vi "Untitled-2SubVI (1).vi"(8 "Array in":u16[][](array[numeric]), 9 "Numeric 2":dbl, 10 "Numeric":dbl, 11 "shuffled array":i32[][](array[numeric])) -> (3 "Array out":u16[][](array[numeric]))   [LabVIEW 2020]
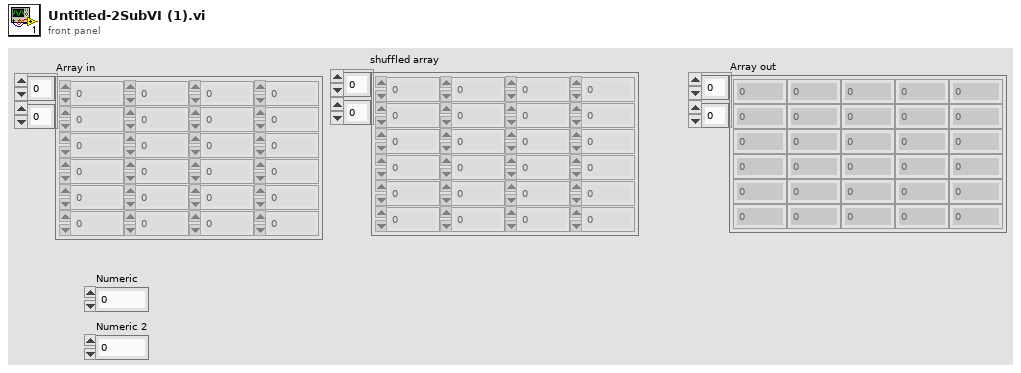
[diagram p1: front panel]
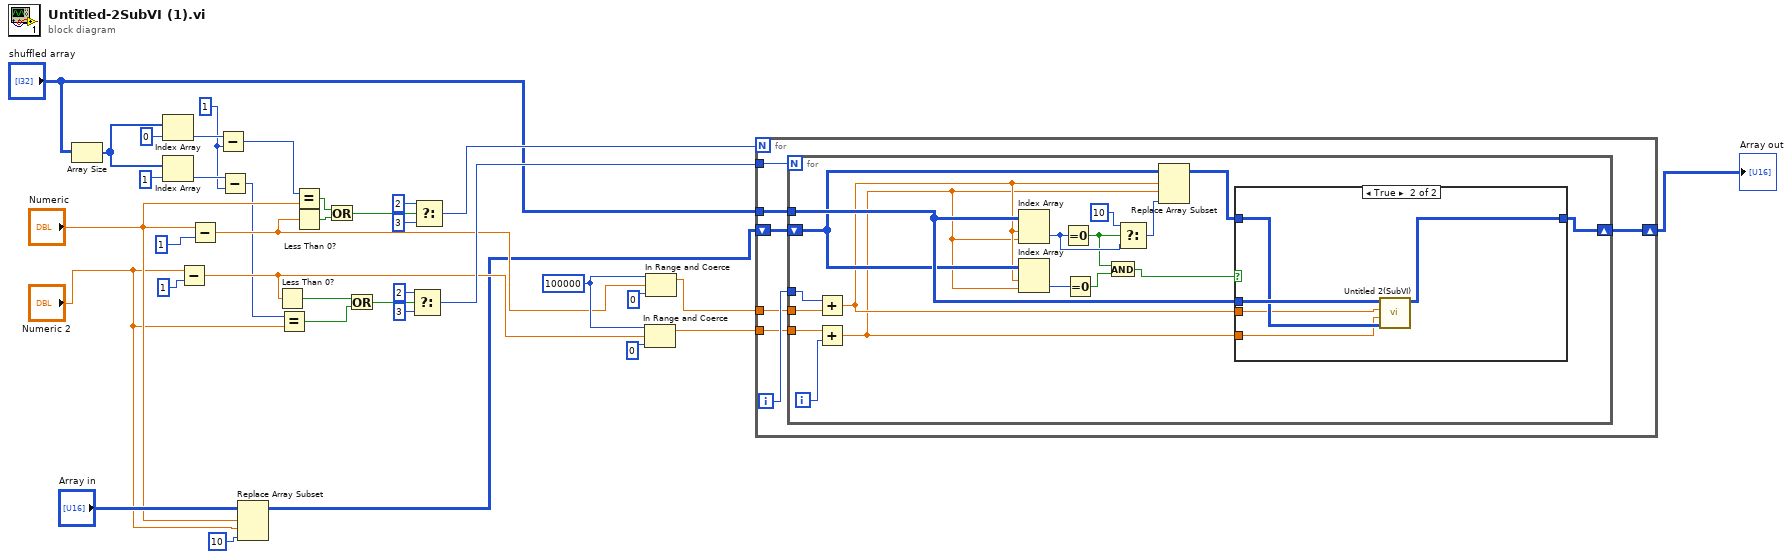
[diagram p0: block diagram]
diagram:
  w3 = 1
  w26 = 100000
  n1 = Array Size(array="shuffled array") -> (size(s)=w16:i32[])
  n2 = Index Array(array=w16, index=0) -> (element=w5:i32)
  n3 = Index Array(array=w16, index=1) -> (element=w4:i32)
  n4 = Subtract(x="Numeric 2", y=1) -> (x-y=w23:dbl)
  n5 = Subtract(x="Numeric", y=1) -> (x-y=w25:dbl)
  n6 = Subtract(x=w5, y=w3) -> (x-y=w2:i32)
  n7 = Subtract(x=w4, y=w3) -> (x-y=w1:i32)
  n8 = Replace Array Subset(array="Array in", new element=10, index (row)="Numeric", index (col)="Numeric 2") -> (w19:u16[][])
  n9 = Less Than 0?(x=w23) -> (x < 0?=w10:bool)
  n10 = Equal?(x=w1, y="Numeric 2") -> (x = y?=w9:bool)
  n11 = Equal?(x=w2, y="Numeric") -> (x = y?=w13:bool)
  n12 = Less Than 0?(x=w25) -> (x < 0?=w14:bool)
  n13 = Or(x=w13, y=w14) -> (x .or. y?=w12:bool)
  n14 = Or(x=w10, y=w9) -> (x .or. y?=w11:bool)
  n15 = Select(t=2, s=w11, f=3) -> (s? t:f=w29:i32)
  n16 = Select(t=2, s=w12, f=3) -> (s? t:f=w30:i32)
  n17 = In Range and Coerce(upper limit=w26, x=w23, lower limit=0) -> (coerced(x)=w21:dbl)  [unwired: 1 out]
  n18 = In Range and Coerce(upper limit=w26, x=w25, lower limit=0) -> (coerced(x)=w22:dbl)  [unwired: 1 out]
  n19 = for {
    N: w30 -> [_]
    tunnel: w29 -> [w42]
    shift-right: [w40] -> w24
    shift-left: w19 -> [w43]
    tunnel: w22 -> [w39]
    tunnel: w21 -> [w38]
    tunnel: "shuffled array" -> [w37]
    i -> [w41]
    n20 = for {
      N: w42 -> [_]
      tunnel: w41 -> [w59]
      shift-right: [w52] -> w40
      shift-left: w43 -> [w50]
      tunnel: w39 -> [w60]
      tunnel: w38 -> [w58]
      tunnel: w37 -> [w51]
      i -> [w57]
      n21 = Add(x=w59, y=w60) -> (x+y=w48:dbl)
      n22 = Add(x=w58, y=w57) -> (x+y=w47:dbl)
      n23 = Index Array(array=w51, index (row)=w48, index (col)=w47) -> (element=w54:i32)
      n24 = Index Array(array=w50, index (row)=w48, index (col)=w47) -> (element=w49:u16)
      n25 = Equal To 0?(x=w54) -> (x = 0?=w45:bool)
      n26 = Equal To 0?(x=w49) -> (x = 0?=w46:bool)
      n27 = And(x=w45, y=w46) -> (x .and. y?=w44:bool)
      n28 = Select(t=10, s=w45, f=w54) -> (s? t:f=w56:i32)
      n29 = Replace Array Subset(array=w50, new element=w56, index (row)=w48, index (col)=w47) -> (w53:u16[][])
      n30 = case shown="True" w44 {
        tunnel: w53 -> [w61 w65]
        tunnel: [w61 w64] -> w52
        tunnel: w51 -> [_ w66]
        tunnel: w48 -> [_ w63]
        tunnel: w47 -> [_ w62]
        frame False {
        }
        frame True {
          n31 = call "Untitled 2(SubVI).vi"("Array in"=w65, "Numeric 2"=w62, "Numeric"=w63, "shuffled array"=w66) -> ("Array out"=w64:u16[][])  [unwired: 7 in]
        }
      }
    }
  }
  "Array out" <- w24
